vi "Save header.vi"(7 "scale info":cluster{"multiplier":sgl, "offset":sgl}[](array[cluster]) {"offset" format="%.2f"; "multiplier" format="%.2f"}, 8 "sample rate":sgl format="%.2f", 9 "channels":T1[](array[typedef]) {"input config" items=["no change", "differential", "ref. single-ended", "non-ref. single-ended", "4-wire"]; "coupling" items=["no change", "DC", "AC", "GND", "internal ref."]; "engineering units" items=["custom...", "V", "Pa", "g", "m/s^2", "m/s", "m", "in/s^2", "in/s", "in"]; "sensor sensitivity (mV/EU)" format="%.2f"; "range(+_)" format="%.2f"}, 10 "file name":string, 11 "data folder":path) -> (3 "file refnum":refnum<file>)   [LabVIEW 2017]
uses:
  <vilib>/addons/Sound and Vibration/Order Analysis/Misc/OAT Channel Setting.ctl
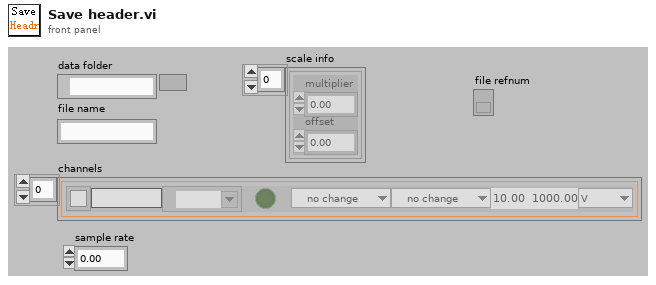
[diagram p1: front panel]
types:
  T1 = typedef "OAT Channel Setting.ctl" = cluster{"color":u32, "name":string, "channel":tag, "coupling":u16, "input config":u16, "range(+_)":sgl, "sensor sensitivity (mV/EU)":dbl, "engineering units":u16, "excitation":bool}
  T2 = enum16{"open", "open or create", "create or replace", "create", "open (read only)"}
  T3 = cluster{"name":string, "multiplier":sgl, "offset":sgl, "sensor sensitivity (mV/EU)":dbl, "engineering units":u16}
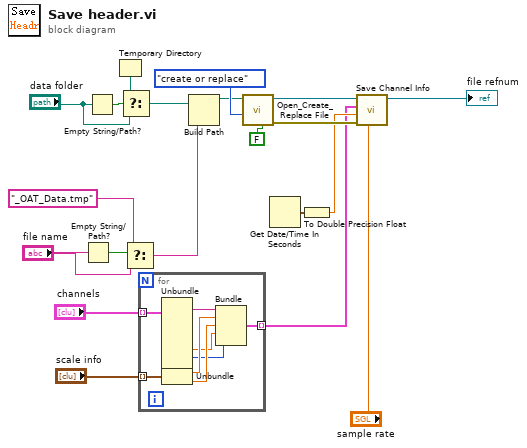
[diagram p0: block diagram]
diagram:
  n1 = Empty String/Path?(string/path="file name") -> (empty?=w10:bool)
  n2 = Empty String/Path?(string/path="data folder") -> (empty?=w11:bool)
  n3 = Temporary Directory() -> (w14:path)
  n4 = Select(t=w14, s=w11, f="data folder") -> (s? t:f=w13:path)
  n5 = Select(t="_OAT_Data.tmp" ("time format string (%c)"), s=w10, f="file name") -> (s? t:f=w8:string)
  n6 = for {
    tunnel: "channels" -> [w28] mode=indexing
    tunnel: [w27] -> w2 mode=indexing
    tunnel: "scale info" -> [w25] mode=indexing
    n7 = Unbundle(w28) -> ("name"=w26:string, "sensor sensitivity (mV/EU)"=w22:dbl, "engineering units"=w21:u16)  [unwired: 6 out]
    n8 = Unbundle(w25) -> ("multiplier"=w24:sgl, "offset"=w23:sgl)
    n9 = Bundle("name"=w26, "multiplier"=w24, "offset"=w23, "sensor sensitivity (mV/EU)"=w22, "engineering units"=w21) -> (w27:T3)  [unwired: 1 in]
  }
  n10 = Build Path(base path=w13, name or relative path=w8) -> (appended path=w18:path)
  n11 = call <vilib>:"Open_Create_Replace File.vi"("advisory dialog? (display:T)"=FALSE, "function (open:0)"=T2."create or replace", "file path"=w18) -> ("error out"=w15:errorcluster, "refnum"=w16:refnum<file>)  [unwired: 5 in, 2 out]
  n12 = Get Date/Time In Seconds() -> (seconds since 1Jan1904=w1:timestamp)
  n13 = To Double Precision Float(number=w1) -> (double precision float=w4:dbl)
  n14 = call <vilib>:"Save Channel Info.vi"("Sample rate"="sample rate", "error in"=w15, "time"=w4, "channel info"=w2, "refnum in"=w16) -> ("refnum out"=→"file refnum":refnum<file>)  [unwired: 5 in, 1 out]
